vi "饼图.vi"() -> ()   [LabVIEW 2012]
uses:
  <vilib>/Math Plots/3D Math Plots/3D Pie/3D Pie XCtrl/3D Pie.xctl
  <vilib>/Math Plots/3D Math Plots/3D Pie/3D Pie Datatype/Public/Plot Helper (Vector).vi
  <vilib>/imath/engines/lvmath2/RunTimeEngine/ErrorHandling/NIMS_Finalize Error.vi
  <vilib>/imath/engines/lvmath2/RunTimeEngine/NodeEndStatement/NIMS_NodeEndStatement_Output.vi
  <instcachedir>/0/NIMS_NodeEndStatement_Output_53EC0D466D134D7ABD903AC30B43404B.lvgen/NIMS_NodeEndStatement_Output_53EC0D466D134D7ABD903AC30B43404B_005.vi
  <vilib>/imath/engines/lvmath2/RunTimeEngine/BuiltInFunctions/rand/NIMS_rand(1,I32).vi
  <vilib>/imath/engines/lvmath2/RunTimeEngine/ErrorHandling/NIMS_Error From Error Code.vi
  <vilib>/imath/engines/lvmath2/RunTimeEngine/BuiltInFunctions/pie/NIMS_pie.vi
  <vilib>/imathl/engines/lvmath/Functions/Error Handling/Create Error.vi
  <vilib>/Math Plots/3D Math Plots/3D Pie/3D Pie Datatype/3D Pie Datatype.lvclass
panel:
  out "3D Pie":refnum<class "3D Plot Datatype.lvclass">[](xcontrol) caption="三维饼图"
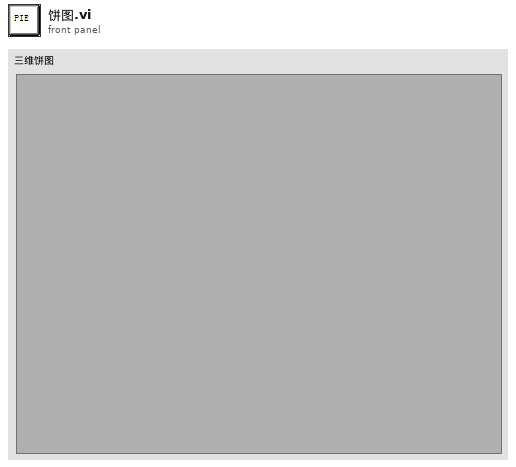
[diagram p1: front panel]
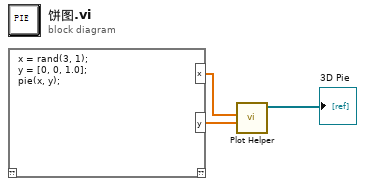
[diagram p0: block diagram]
diagram:
  n1 = mathscript code="x = rand(3, 1);\ny = [0, 0, 1.0];\npie(x, y);"() -> ("x"=w2:dbl[], "y"=w1:dbl[])  [unwired: 1 in, 1 out]
  n2 = call-poly <vilib>:"Plot Helper.vi"("offset vector"=w1, "x vector"=w2) -> ("3D Plot lvclass Array out"=→"3D Pie":refnum<class "3D Plot Datatype.lvclass">[])  [unwired: 1 in, 8 out]
